vi "Configure Multitone (Custom).vi"(0 "template configuration":refnum<class "SV Signal.lvclass">, 1 "overall amplitude":dbl=1.0, 5 "frequencies [Hz]":dbl[](array[numeric])=[100.0, 200.0, 300.0], 7 "amplitudes":dbl[](array[numeric])=[1.0, 1.0, 1.0], 9 "phases [deg]":dbl[](array[numeric])=[0.0, 90.0, 270.0], 11 "error in (no error)":errorcluster) -> (4 "signal configuration":refnum<class "SV Multitone.lvclass">, 6 "tones":T1(array[cluster]), 15 "error out":errorcluster)   [LabVIEW 2017, in "SV Multitone.lvclass"]
doc: "Configures a user-defined test signal. Wire the outputs to SV Signal (waveform) VI to generate the test signal, or wire to SV Signal Property Node to configure additional parameters before wiring to the SV Signal (waveform) VI."
uses:
  <vilib>/addons/_NISVFA/_Generation/Signal Generation/SV Multitone/SV Multitone.lvclass
  C:/Program Files (x86)/National Instruments/LabVIEW 2017/vi.lib/addons/_NISVFA/_Generation/Signal Generation/SV Signal/SV Signal.lvclass
  <vilib>/addons/_NISVFA/_Generation/Signal Generation/SV Signal/SV Signal.lvclass
  <vilib>/addons/_NISVFA/_Generation/Signal Generation/SV Multitone/SV Multitone.lvclass/SV Multitone.ctl
  <vilib>/addons/_NISVFA/_Generation/Signal Generation/SV Signal/Read Sample Rate.vi
  <vilib>/addons/_NISVFA/_Generation/Signal Generation/SV Signal/Read Measurement Duration.vi
  <vilib>/addons/_NISVFA/_Generation/Signal Generation/SV Signal/Write Measurement Duration.vi
  <vilib>/addons/_NISVFA/_Generation/Signal Generation/SV Signal/Write Sample Rate.vi
  <vilib>/addons/_NISVFA/_Shared subVIs/Common/svc_Is X a Factor of Y.vi
  <vilib>/Analysis/NI_AALBase.lvlib
  <vilib>/measure/NI_MAPro.lvlib
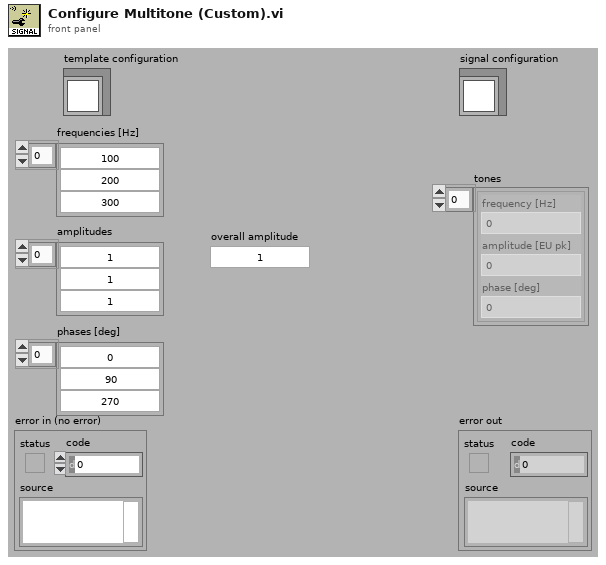
[diagram p1: front panel]
types:
  T1 = cluster{"frequency [Hz]":dbl, "amplitude [EU pk]":dbl, "phase [deg]":dbl}[]
  T2 = cluster{"frequency [Hz]":dbl, "amplitude [EU pk]":dbl, "phase (deg)":dbl}
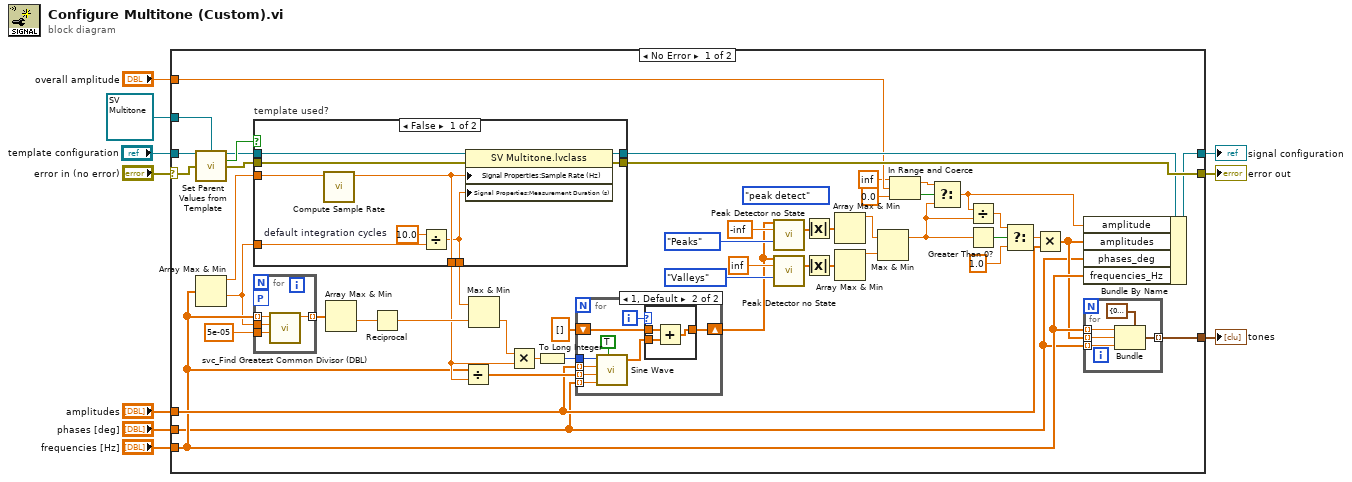
[diagram p0: block diagram]
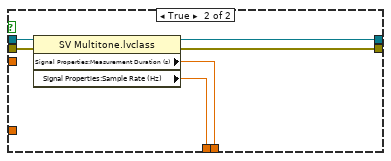
[diagram p2: hidden frame]
diagram:
  n1 = case shown="No Error" "error in (no error)" {
    selector: "error in (no error)" -> [w28 w97]
    tunnel: [w59 w97] -> w9
    tunnel: [w35 w98] -> w3
    tunnel: refnum<class "SV Multitone.lvclass"> refnum ("Multitone in") -> [w27 w98]
    tunnel: "frequencies [Hz]" -> [w15 _]
    tunnel: "amplitudes" -> [w37 _]
    tunnel: "phases [deg]" -> [w13 _]
    tunnel: "overall amplitude" -> [w23 _]
    tunnel: "template configuration" -> [w29 _]
    tunnel: [w12 _] -> w1
    frame No Error {
      (unwired) enum16{"max absolute value", "peak detect"}."peak detect" ("scaling method")
      n2 = call-dynamic "Set Parent Values from Template.vi"("template configuration"=w29, "signal configuration in"=w27, "error in (no error)"=w28) -> ("signal configuration out"=w24:refnum<class "SV Multitone.lvclass">, "template used?"=w25:bool, "error out"=w17:errorcluster)  [unwired: 10 in]
      n3 = Array Max & Min(array=w15) -> (max value=w58:dbl, min value=w11:dbl)  [unwired: 2 out]
      n4 = case "template used?" shown="False" w25 {
        tunnel: w24 -> [w73 w79]
        tunnel: [w72 w76] -> w59
        tunnel: w58 -> [w71 _]
        tunnel: [w70 w75] -> w40
        tunnel: [w69 w77] -> w36
        tunnel: w17 -> [w68 w78]
        tunnel: [w67 w74] -> w26
        tunnel: w11 -> [w65 _]
        frame False {
          w66 = 10.0  # default integration cycles
          n5 = call <vilib>:"Compute Sample Rate.vi"("maximum frequency [Hz]"=w71) -> ("sample rate [Hz]"=w70:dbl)  [unwired: 10 in]
          n6 = Divide(x=w66, y=w65) -> (x/y=w67:dbl)
          n7 = property class="SV Multitone.lvclass"(reference=w73, error in=w68, "Signal Properties:Sample Rate (Hz)"=w70, "Signal Properties:Measurement Duration (s)"=w67) -> (reference out=w69:refnum<class "SV Multitone.lvclass">, error out=w72:errorcluster)
        }
        frame True {
          n8 = property class="SV Multitone.lvclass"(reference=w79, error in=w78) -> (reference out=w77:refnum<class "SV Multitone.lvclass">, error out=w76:errorcluster, "Signal Properties:Measurement Duration (s)"=w74:dbl, "Signal Properties:Sample Rate (Hz)"=w75:dbl)
        }
      }
      n9 = for {
        tunnel: w15 -> [w83] mode=indexing
        tunnel: w11 -> [w82]
        tunnel: [w81] -> w55 mode=indexing
        workers-P: _ -> [_]
        tunnel: 5e-05 ("tolerance") -> [w80]
        n10 = call <vilib>:"svc_Find Greatest Common Divisor (DBL).vi"("tolerance"=w80, "y"=w82, "x"=w83) -> ("gcd(x,y)"=w81:dbl)  [unwired: 8 in]
      }
      n11 = Array Max & Min(array=w55) -> (min value=w54:dbl)  [unwired: 3 out]
      n12 = Reciprocal(x=w54) -> (1/x=w42:dbl)
      n13 = Divide(x=w15, y=w40) -> (x/y=w56:dbl[])
      n14 = Max & Min(x=w26, y=w42) -> (min(x,y)=w41:dbl)  [unwired: 1 out]
      n15 = Multiply(x=w41, y=w40) -> (x*y=w39:dbl)
      n16 = To Long Integer(number=w39) -> (32bit integer=w38:i32)
      n17 = for {
        tunnel: w38 -> [w92]
        tunnel: w37 -> [w90] mode=indexing
        tunnel: w13 -> [w89] mode=indexing
        shift-right: [w86] -> w43
        shift-left: dbl[] [] ("sine wave") -> [w85]
        tunnel: w56 -> [w84] mode=indexing
        i -> [w88]
        n18 = call <vilib>:"Sine Wave.vi"("samples"=w92, "amplitude"=w90, "frequency"=w84, "phase in"=w89, "reset phase"=TRUE ("coerce frequencies?")) -> ("sine wave"=w87:dbl[])  [unwired: 2 out]
        n19 = case shown="1, Default" w88 {
          tunnel: w87 -> [w93 w96]
          tunnel: [w93 w95] -> w86
          tunnel: w85 -> [_ w94]
          frame 0 {
          }
          frame 1, Default {
            n20 = Add(x=w94, y=w96) -> (x+y=w95:dbl[])
          }
        }
      }
      n21 = call <vilib>:"Peak Detector no State.vi"("X"=w43, "threshold"=-inf, "peaks/valleys"=enum32{"Peaks", "Valleys"}."Peaks") -> ("Amplitudes"=w48:dbl[])  [unwired: 5 in, 7 out]
      n22 = call <vilib>:"Peak Detector no State.vi"("X"=w43, "threshold"=inf, "peaks/valleys"=enum32{"Peaks", "Valleys"}."Valleys") -> ("Amplitudes"=w49:dbl[])  [unwired: 5 in, 7 out]
      n23 = Absolute Value(x=w48) -> (abs(x)=w46:dbl[])
      n24 = Absolute Value(x=w49) -> (abs(x)=w47:dbl[])
      n25 = Array Max & Min(array=w46) -> (max value=w45:dbl)  [unwired: 3 out]
      n26 = Array Max & Min(array=w47) -> (max value=w44:dbl)  [unwired: 3 out]
      n27 = Max & Min(x=w45, y=w44) -> (max(x,y)=w18:dbl)  [unwired: 1 out]
      n28 = In Range and Coerce(upper limit=inf, x=w23, lower limit=0.0) -> (coerced(x)=w19:dbl, In Range?=w20:bool)
      n29 = Select(t=w19, s=w20, f=w18) -> (s? t:f=w16:dbl)
      n30 = Divide(x=w16, y=w18) -> (x/y=w32:dbl)
      n31 = Greater Than 0?(x=w18) -> (x > 0?=w34:bool)
      n32 = Select(t=w32, s=w34, f=1.0) -> (s? t:f=w31:dbl)
      n33 = Multiply(x=w31, y=w37) -> (x*y=w14:dbl[])
      n34 = Bundle By Name(cluster=w36, "amplitude"=w16, "amplitudes"=w14, "phases_deg"=w13, "frequencies_Hz"=w15) -> (w35:refnum<class "SV Multitone.lvclass">)
      n35 = for {
        tunnel: w15 -> [w64] mode=indexing
        tunnel: w14 -> [w63] mode=indexing
        tunnel: w13 -> [w62] mode=indexing
        tunnel: [w60] -> w12 mode=indexing
        n36 = Bundle(cluster=T2 {"frequency [Hz]"=0.0, "amplitude [EU pk]"=0.0, "phase (deg)"=0.0} ("tone"), "frequency [Hz]"=w64, "amplitude [EU pk]"=w63, "phase (deg)"=w62) -> (w60:T2)
      }
    }
    frame Error {
    }
  }
  "error out" <- w9
  "signal configuration" <- w3
  "tones" <- w1
